vi "util-io-csv-save.vi"(8 "error out":errorcluster, 10 "file path (dialog if empty)":path, 11 "IO Nodes":T1[](array[typedef]) {"calibration"."Y" format="%#.3f"; "calibration"."X" format="%#.3f"; "ADDR" format="%04d"}) -> (0 "error out":errorcluster)   [LabVIEW 2024]
uses:
  controls/IONode.ctl
  controls/type.address.ctl
  controls/enum.io.type.ctl
  controls/enum.io.mode.ctl
  controls/typeXyPoint.ctl
  <vilib>/Utility/file.llb/Write Delimited Spreadsheet (string).vi
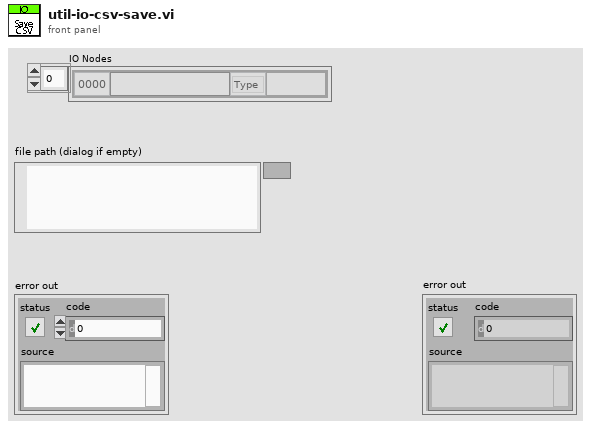
[diagram p1: front panel]
types:
  T1 = typedef "IONode.ctl" = cluster{"ADDR":T2, "Label":string, "Type":T3, "Mode":T4, "Value":string, "Tags":string, "calibration":T5[]}
  T2 = typedef "type.address.ctl" = u16
  T3 = typedef "enum.io.type.ctl" = enum16{"Type", "DI", "DO", "AI", "AO", "VL", "BUF"}
  T4 = typedef "enum.io.mode.ctl" = enum16{"Mode", "RIO", "SIM"}
  T5 = typedef "typeXyPoint.ctl" = cluster{"X":dbl, "Y":dbl}
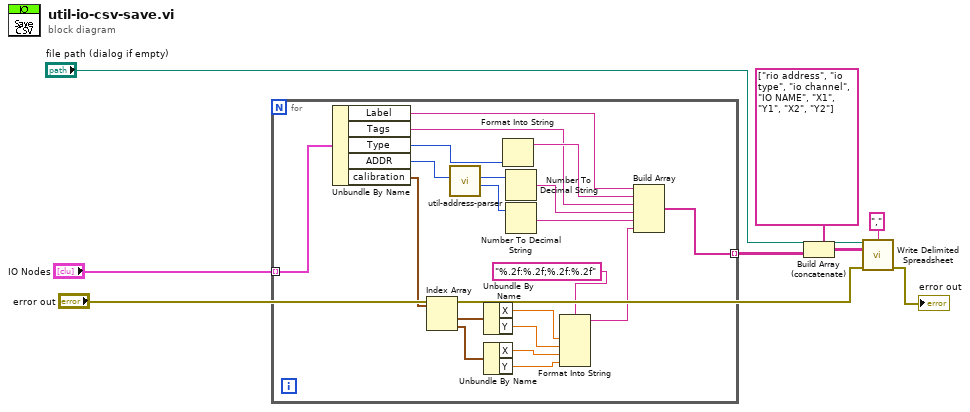
[diagram p0: block diagram]
diagram:
  n1 = for {
    tunnel: "IO Nodes" -> [w28] mode=indexing
    tunnel: [w16] -> w6 mode=indexing
    n2 = Unbundle By Name(w28) -> ("Label"=w23:string, "Tags"=w18:string, "Type"=w17:T3, "ADDR"=w21:T2, "calibration"=w15:T5[])
    n3 = Index Array(array=w15) -> (element #1=w25:T5, element #2=w24:T5)  [unwired: 2 in]
    n4 = call "util-address-parser.vi"("ADDR 2"=w21) -> ("Channel"=w26:u8, "Address"=w27:u8)  [unwired: 9 in]
    n5 = Unbundle By Name(w25) -> ("X"=w13:dbl, "Y"=w12:dbl)
    n6 = Unbundle By Name(w24) -> ("X"=w11:dbl, "Y"=w10:dbl)
    n7 = Format Into String(w17) -> (resulting string=w22:string)  [unwired: 3 in, 1 out]
    n8 = Number To Decimal String(number=w27) -> (decimal integer string=w20:string)  [unwired: 1 in]
    n9 = Number To Decimal String(number=w26) -> (decimal integer string=w19:string)  [unwired: 1 in]
    n10 = Format Into String(format string="%.2f:%.2f;%.2f:%.2f", w13, w12, w11, w10) -> (resulting string=w9:string)  [unwired: 2 in, 1 out]
    n11 = Build Array(w23, w22, w18, w20, w19, w9) -> (w16:string[])
  }
  n12 = Build Array (concatenate)(string[] ["rio address", "io type", "io channel", "IO NAME", "X1", "Y1", "X2", "Y2"] ("headers"), w6) -> (w3:string[][])
  n13 = call-poly <vilib>:"Write Delimited Spreadsheet.vi"("file path (dialog if empty)"="file path (dialog if empty)", "2D data"=w3, "error in (no error)"="error out", "delimiter (\\t)"="," ("delimiter (\\t)")) -> ("error out"=→"error out":errorcluster)  [unwired: 10 in, 1 out]
